vi "Burster 1427 Set RTD b.vi"(1 "Error In":errorcluster={"status"=TRUE, "code"=0, "source"=""}, 2 "RTD Setting":dbl, 3 "VISA resource name":refnum<visa-resource-name>) -> (0 "Error Out":errorcluster)   [LabVIEW 2013]
uses:
  <vilib>/Instr/_visa.llb/VISA Configure Serial Port (Instr).vi
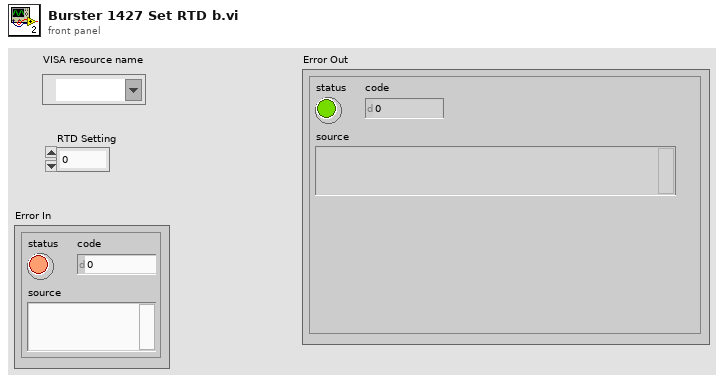
[diagram p1: front panel]
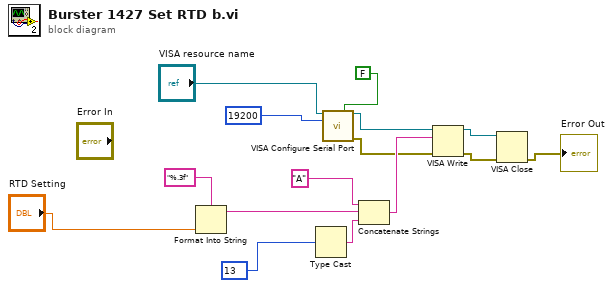
[diagram p0: block diagram]
diagram:
  n1 = Format Into String(format string="%.3f", "RTD Setting") -> (resulting string=w12:string)  [unwired: 2 in, 1 out]
  n2 = Type Cast(x=u8 13) -> (*(type *) &x=w2:string)  [unwired: 1 in]
  n3 = call-poly "VISA Configure Serial Port"("VISA resource name"="VISA resource name", "Enable Termination\nChar (T)"=FALSE, "baud rate (9600)"=19200) -> ("VISA resource name out"=w8:refnum<visa-resource-name>, "error out"=w7:errorcluster)  [unwired: 11 in]
  n4 = Concatenate Strings("A", w12, w2) -> (w11:string)
  n5 = VISA Write(VISA resource name=w8, write buffer=w11, error in (no error)=w7) -> (VISA resource name out=w6:refnum<visa-resource-name>, error out=w5:errorcluster)  [unwired: 1 out]
  n6 = VISA Close(VISA resource name=w6, error in (no error)=w5) -> (error out=→"Error Out":errorcluster)
